vi "Create Sequences for Test Configuration.vi"() -> (3 "Lines":T1[](array[typedef]))   [LabVIEW 2015, in "Sequencer Module tests.lvlib"]
uses:
  Sequencer Module tests.lvlib
  module/configuration/Line.ctl
  classes/Sequence/Config/Sequence Config.lvclass
  module/configuration/Sequencer Module configuration.lvclass
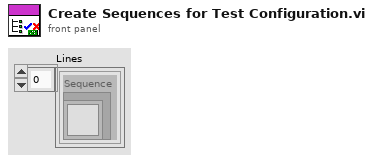
[diagram p1: front panel]
types:
  T1 = typedef "Sequencer Module configuration.lvclass/Line.ctl" = cluster{"Sequence":refnum<class "Sequence Config.lvclass">}
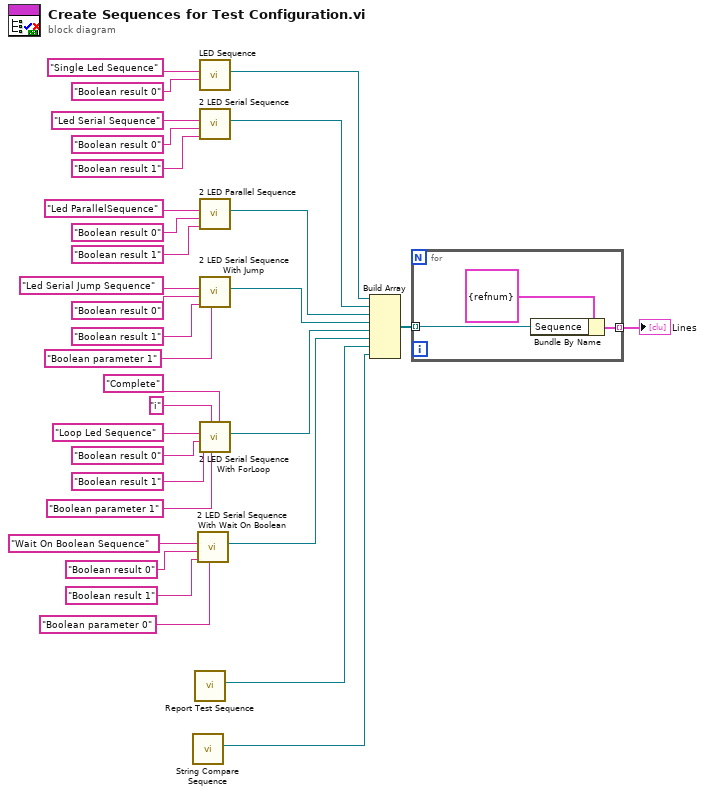
[diagram p0: block diagram]
diagram:
  n1 = call "String Compare Sequence.vi"() -> ("Sequence"=w31:refnum<class "Sequence Config.lvclass">)  [unwired: 11 in]
  n2 = call "Report Test Sequence.vi"() -> ("Sequence"=w30:refnum<class "Sequence Config.lvclass">)  [unwired: 11 in]
  n3 = call "2 LED Serial Sequence With Wait On Boolean.vi"("Jump Tag Name"="Boolean parameter 0" ("Tag Name"), "Tag Name 2"="Boolean result 1" ("Tag Name"), "Tag Name 1"="Boolean result 0" ("Tag Name"), "Name"="Wait On Boolean Sequence") -> ("Sequence out"=w29:refnum<class "Sequence Config.lvclass">)  [unwired: 7 in]
  n4 = call "LED Sequence.vi"("Tag Name"="Boolean result 0", "Name"="Single Led Sequence") -> ("Sequence out"=w20:refnum<class "Sequence Config.lvclass">)  [unwired: 9 in]
  n5 = call "2 LED Serial Sequence.vi"("Tag Name 2"="Boolean result 1" ("Tag Name"), "Tag Name 1"="Boolean result 0" ("Tag Name"), "Name"="Led Serial Sequence") -> ("Sequence out"=w21:refnum<class "Sequence Config.lvclass">)  [unwired: 8 in]
  n6 = call "2 LED Parallel Sequence.vi"("Tag Name 2"="Boolean result 1" ("Tag Name"), "Tag Name 1"="Boolean result 0" ("Tag Name"), "Name"="Led ParallelSequence") -> ("Sequence out"=w24:refnum<class "Sequence Config.lvclass">)  [unwired: 8 in]
  n7 = call "2 LED Serial Sequence With Jump.vi"("Jump Tag Name"="Boolean parameter 1" ("Tag Name"), "Tag Name 2"="Boolean result 1" ("Tag Name"), "Tag Name 1"="Boolean result 0" ("Tag Name"), "Name"="Led Serial Jump Sequence") -> ("Sequence out"=w22:refnum<class "Sequence Config.lvclass">)  [unwired: 7 in]
  n8 = call "2 LED Serial Sequence With ForLoop.vi"("Completed Tag name"="Complete", "Jump Tag Name"="Boolean parameter 1" ("Tag Name"), "Iteration Tag Name"="i", "Tag Name 2"="Boolean result 1" ("Tag Name"), "Tag Name 1"="Boolean result 0" ("Tag Name"), "Name"="Loop Led Sequence") -> ("Sequence out"=w23:refnum<class "Sequence Config.lvclass">)  [unwired: 5 in]
  n9 = Build Array(w20, w21, w24, w22, w23, w29, w30, w31) -> (w25:refnum<class "Sequence Config.lvclass">[])
  n10 = for {
    tunnel: [w35] -> w13 mode=indexing
    tunnel: w25 -> [w33] mode=indexing
    n11 = Bundle By Name(cluster=T1 {"Sequence"=refnum} ("Line"), "Sequence"=w33) -> (w35:T1)
  }
  "Lines" <- w13
